vi "SetLaserParameters.vi"(0 "FrameRangeEnd (0-100, end-start >= 25)":i32 min=0 max=100 step=1, 1 "FrameRangeStart (0-100, end-start >= 25)":i32 min=0 max=100 step=1, 2 "LaserFringeCodingMode (Fast Accurate Reflective)":u8(ring) items=["Fast", "Accurate", "Reflective"], 5 "PowerLevel (50-100)":i32 min=0 max=100 step=1, 6 "FramePartitionCount (1-4)":i32=1 min=1 max=4 step=1, 7 "error in (no error)":errorcluster, 8 "Camera Reference in":refnum<k24>) -> (3 "error out":errorcluster, 4 "Camera Reference out":refnum<k24>)   [LabVIEW 2023]
uses:
  C:/Mech-Mind/Mech-Eye SDK-2.5.0-b5-dev-01-03/API/dll/net48/MechEyeApiNet.dll
  dll/net48/MechEyeApiNet.dll
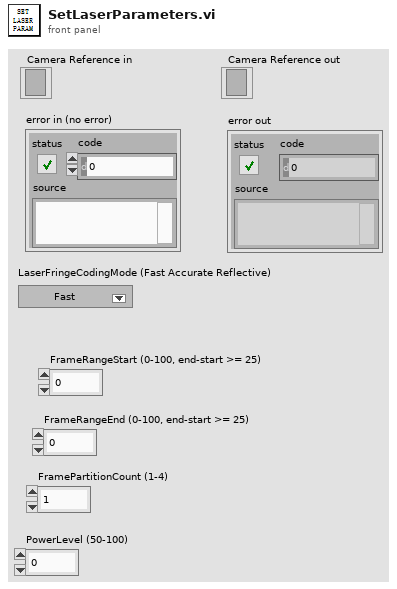
[diagram p1: front panel]
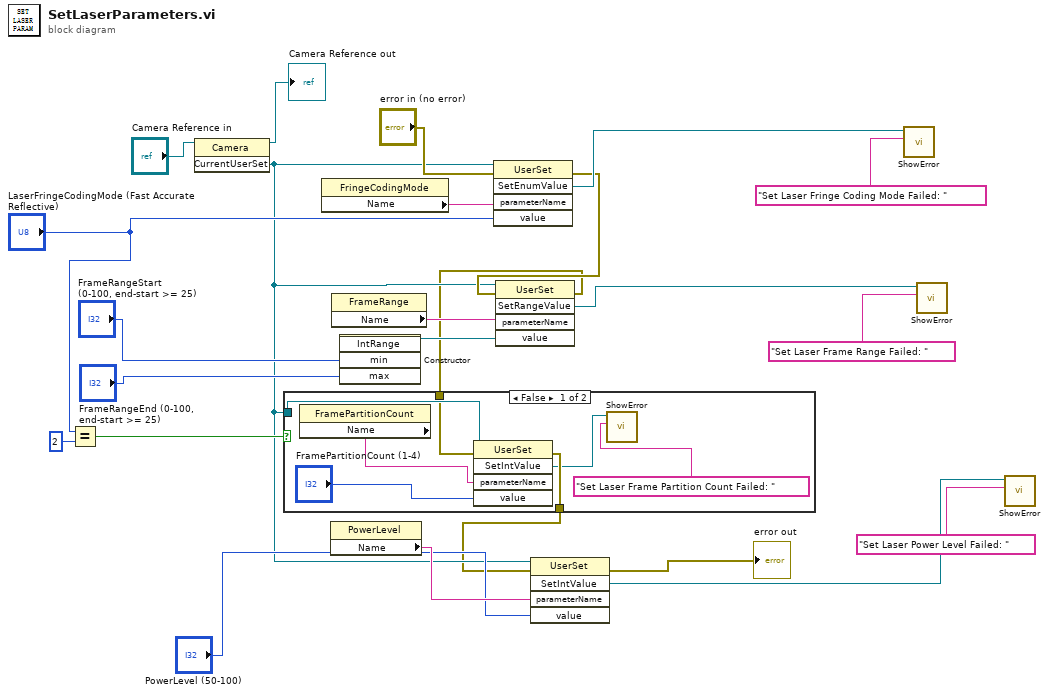
[diagram p0: block diagram]
diagram:
  n1 = Equal?(x="LaserFringeCodingMode (Fast Accurate Reflective)", y=2) -> (x = y?=w4:bool)
  n2 = invoke class="Camera" method="CurrentUserSet"(reference="Camera Reference in") -> (reference out=→"Camera Reference out":refnum<k24>, "CurrentUserSet"=w3:refnum<k24>)  [unwired: 2 in, 1 out]
  n3 = property class="FringeCodingMode"() -> ("Name"=w22:string)  [unwired: 2 in, 2 out]
  n4 = property class="PowerLevel"() -> ("Name"=w17:string)  [unwired: 2 in, 2 out]
  n5 = property class="FrameRange"() -> ("Name"=w19:string)  [unwired: 2 in, 2 out]
  n6 = constructor class="IntRange"("min"="FrameRangeStart (0-100, end-start >= 25)", "max"="FrameRangeEnd (0-100, end-start >= 25)") -> (reference out=w18:refnum<k24>)  [unwired: 3 in, 4 out]
  n7 = invoke class="UserSet" method="SetEnumValue"(reference=w3, error in="error in (no error)", "parameterName"=w22, "value"="LaserFringeCodingMode (Fast Accurate Reflective)") -> (error out=w16:errorcluster, "SetEnumValue"=w21:refnum<k24>)  [unwired: 1 in, 3 out]
  n8 = invoke class="UserSet" method="SetRangeValue"(reference=w3, error in=w16, "parameterName"=w19, "value"=w18) -> (error out=w2:errorcluster, "SetRangeValue"=w10:refnum<k24>)  [unwired: 1 in, 3 out]
  n9 = case shown="False" w4 {
    tunnel: w3 -> [w31 _]
    tunnel: w2 -> [w30 w32]
    tunnel: [w27 w32] -> w1
    frame False {
      n10 = property class="FramePartitionCount"() -> ("Name"=w29:string)  [unwired: 2 in, 2 out]
      n11 = invoke class="UserSet" method="SetIntValue"(reference=w31, error in=w30, "parameterName"=w29, "value"="FramePartitionCount (1-4)") -> (error out=w27:errorcluster, "SetIntValue"=w26:refnum<k24>)  [unwired: 1 in, 3 out]
      n12 = call "ShowError.vi"("String"="Set Laser Frame Partition Count Failed: ", "MMind.Eye.ErrorStatus"=w26) -> ()  [unwired: 10 in]
    }
    frame True {
    }
  }
  n13 = invoke class="UserSet" method="SetIntValue"(reference=w3, error in=w1, "parameterName"=w17, "value"="PowerLevel (50-100)") -> (error out=→"error out":errorcluster, "SetIntValue"=w8:refnum<k24>)  [unwired: 1 in, 3 out]
  n14 = call "ShowError.vi"("String"="Set Laser Fringe Coding Mode Failed: ", "MMind.Eye.ErrorStatus"=w21) -> ()  [unwired: 10 in]
  n15 = call "ShowError.vi"("String"="Set Laser Frame Range Failed: ", "MMind.Eye.ErrorStatus"=w10) -> ()  [unwired: 10 in]
  n16 = call "ShowError.vi"("String"="Set Laser Power Level Failed: ", "MMind.Eye.ErrorStatus"=w8) -> ()  [unwired: 10 in]
